vi "Control Squared Objective Function.vi"(9 "Control":dbl[][](array[numeric]), 11 "Time":dbl[](array[numeric])) -> (3 "Objective Func":dbl)   [LabVIEW 2020]
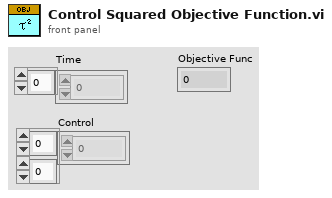
[diagram p1: front panel]
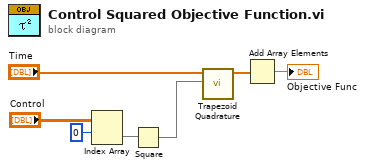
[diagram p0: block diagram]
diagram:
  n1 = Index Array(array="Control", index (row)=0) -> (element=w5:dbl[])  [unwired: 1 in]
  n2 = Square(x=w5) -> (x^2=w4:dbl[])
  n3 = call "Trapezoid Quadrature.vi"("Array"=w4, "Time"="Time") -> ("Result"=w1:dbl[])  [unwired: 9 in]
  n4 = Add Array Elements(numeric array=w1) -> (sum=→"Objective Func":dbl)
